vi "Manual Cartesian Displacement Offset.vi"(8 "error in":errorcluster, 9 "Cartesian Displacements":dbl[](array[numeric]), 10 "Dataset Source":T1, 11 "Is Command":bool) -> (0 "error out":errorcluster)   [LabVIEW 2013]
uses:
  Global Data/Transactions/Dataset Source.ctl
  Data Access Objects/Metadata/Persistant DAO Actions.ctl
  Global Data/Transactions/Dataset Transaction Id.ctl
  Global Data/Transactions/Dataset Type.ctl
  Apps/Yes No Button.ctl
  LbcbConversions/LBCB_Conversions_Actions.ctl
  Data Access Objects/Metadata/DAO Actions with Remove.ctl
  Data Access Objects/Metadata/LBCB Number.ctl
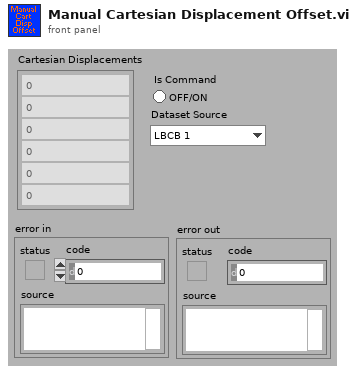
[diagram p1: front panel]
types:
  T1 = typedef "Dataset Source.ctl" = enum16{"LBCB 1", "LBCB 2", "Combined", "External Sensors"}
  T2 = typedef "Dataset Type.ctl" = enum16{"LVDT", "Load Cell", "Actuator Command", "Servo Error", "Displacement Command", "Displacement", "Force"}
  T3 = typedef "DAO Actions with Remove.ctl" = enum16{"Init", "Get", "Set", "Remove"}
  T4 = typedef "LBCB_Conversions_Actions.ctl" = enum16{"A2C", "C2A", "Set Log Filename", "Init"}
  T5 = typedef "Dataset Transaction Id.ctl" = cluster{"Dataset Source":T1, "Dataset Type":T2, "Hold":T6, "Volts":T6, "Tag":string}
  T6 = typedef "Yes No Button.ctl" = bool
  T7 = typedef "Persistant DAO Actions.ctl" = enum16{"Init", "Get", "Set", "Load", "Save"}
  T8 = typedef "LBCB Number.ctl" = enum16{"LBCB1", "LBCB2"}
  T9 = typedef "LBCB Settings.ctl" = cluster{"Size":T10, "Type":T11}
  T10 = typedef "LBCB Size.ctl" = enum16{"1/5th-scale LBCB", "Full-scale LBCB", "Portable LBCB", "Mid-Scale LBCB"}
  T11 = typedef "LBCB Type.ctl" = enum16{"X Actuators On The Left", "X Actuators On The Right"}
  T12 = typedef "LBCB Position.ctl" = cluster{"Motion Center":dbl[], "Transformation Matrix":dbl[][]}
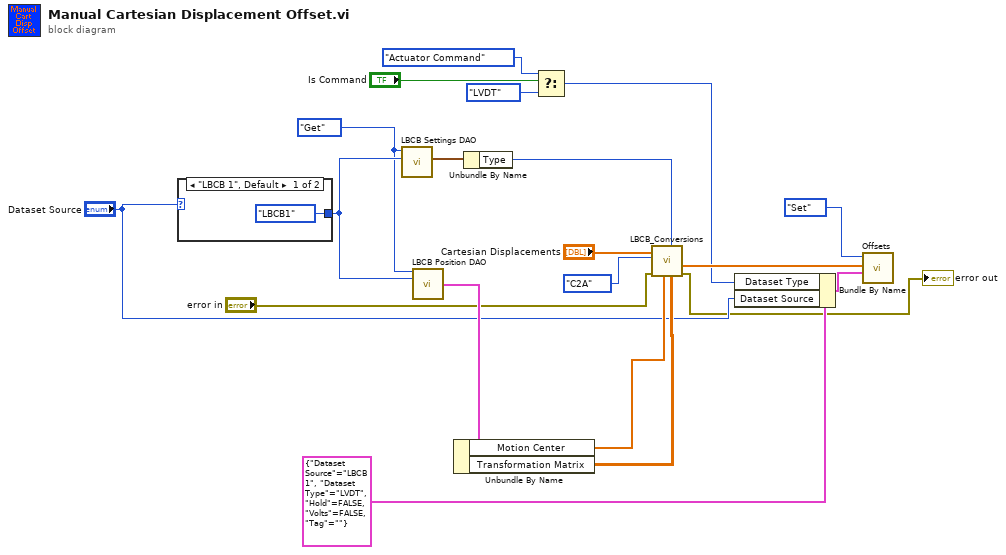
[diagram p0: block diagram]
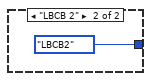
[diagram p2: hidden frame]
diagram:
  w5 = Persistant_DAO_Actions."Get" ("LBCB Settings Actions")
  n1 = case shown="\"LBCB 1\", Default" "Dataset Source" {
    tunnel: [LBCB_Number."LBCB1" ("LBCB Number") LBCB_Number."LBCB2" ("LBCB Number")] -> w10
    frame "LBCB 1", Default {
    }
    frame "LBCB 2" {
    }
  }
  n2 = call "LBCB Settings DAO.vi"("LBCB Number"=w10, "Actions"=w5) -> ("LBCB Setting Out"=w6:T9)  [unwired: 7 in, 2 out]
  n3 = call "LBCB Position DAO.vi"("LBCB Settings Actions"=w5, "LBCB Number"=w10) -> ("LBCB Position Output"=w20:T12)  [unwired: 11 in, 2 out]
  n4 = Unbundle By Name(w20) -> ("Motion Center"=w18:dbl[], "Transformation Matrix"=w19:dbl[][])
  n5 = Unbundle By Name(w6) -> ("Type"=w7:T11)
  n6 = Select(t=Dataset_Type."Actuator Command" ("Dataset Type"), s="Is Command", f=Dataset_Type."LVDT") -> (s? t:f=w1:T2)
  n7 = call "LBCB_Conversions.vi"("Transformation Matrix"=w19, "Type"=w7, "Motion Center"=w18, "error in (no error)"="error in", "Conversion Type"=LBCB_Conversions_Actions."C2A", "Input"="Cartesian Displacements") -> ("error out"=→"error out":errorcluster, "Output"=w14:dbl[])  [unwired: 4 in]
  n8 = Bundle By Name(cluster=T5 {"Dataset Source"=enum."LBCB 1", "Dataset Type"=enum."LVDT", "Hold"=FALSE, "Volts"=FALSE, "Tag"=""} ("Dataset Trans Id"), "Dataset Type"=w1, "Dataset Source"="Dataset Source") -> (w16:T5)
  n9 = call "Offsets.vi"("Dataset Trans Id"=w16, "Data In"=w14, "DAO Actions"=DAO_Actions_with_Remove."Set") -> ()  [unwired: 6 in, 3 out]
